vi "SetVoltage.vi"(3 "Voltage":dbl format="%.3f", 4 "error in":errorcluster, 5 "connection ID":refnum<k5>) -> (0 "False":bool, 1 "error out":errorcluster, 2 "connection ID out":refnum<k5>)   [LabVIEW 2013]
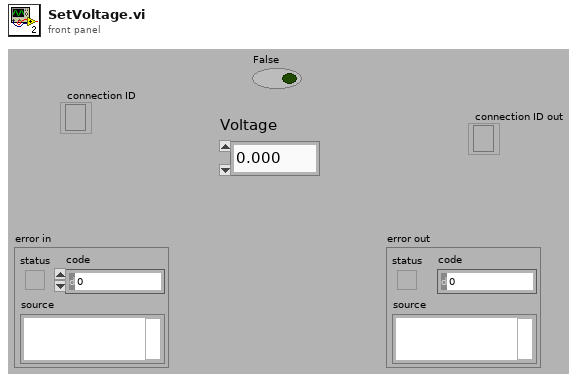
[diagram p1: front panel]
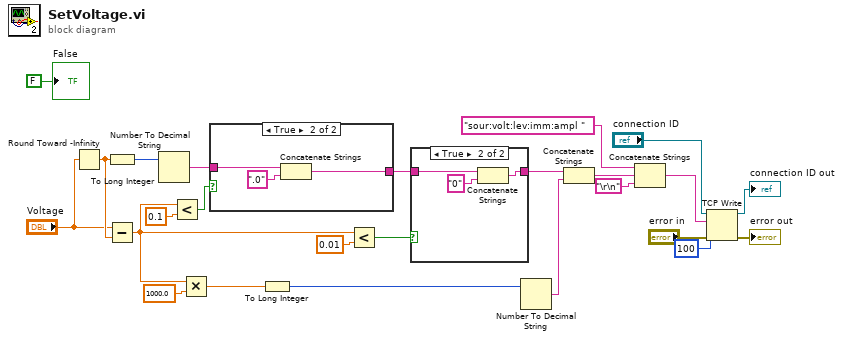
[diagram p0: block diagram]
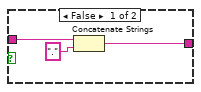
[diagram p3: hidden frame]
diagram:
  n1 = Round Toward -Infinity(1:"Voltage") -> (0:w17:dbl)
  n2 = To Long Integer(number=w17) -> (32bit integer=w15:i32)
  n3 = Subtract(x="Voltage", y=w17) -> (x-y=w10:dbl)
  n4 = Number To Decimal String(number=w15) -> (decimal integer string=w8:string)  [unwired: 1 out]
  n5 = Less?(x=w10, y=0.1) -> (x < y?=w9:bool)
  n6 = Multiply(x=w10, y=1000.0) -> (x*y=w18:dbl)
  n7 = case shown="True" w9 {
    tunnel: w8 -> [w27 w30]
    tunnel: [w26 w29] -> w6
    frame False {
      n8 = Concatenate Strings(w27, "." ("string")) -> (w26:string)
    }
    frame True {
      n9 = Concatenate Strings(w30, ".0" ("string")) -> (w29:string)
    }
  }
  n10 = To Long Integer(number=w18) -> (32bit integer=w16:i32)
  n11 = Less?(x=w10, y=0.01) -> (x < y?=w7:bool)
  n12 = case shown="True" w7 {
    tunnel: w6 -> [w32 w34]
    tunnel: [w32 w33] -> w5
    frame False {
    }
    frame True {
      n13 = Concatenate Strings(w34, "0" ("string")) -> (w33:string)
    }
  }
  n14 = Number To Decimal String(number=w16) -> (decimal integer string=w14:string)  [unwired: 1 out]
  n15 = Concatenate Strings(w5, w14) -> (w4:string)
  n16 = Concatenate Strings("sour:volt:lev:imm:ampl " ("data in"), w4, "\r\n") -> (w23:string)
  n17 = TCP Write(connection ID="connection ID", data in=w23, error in (no error)="error in", 9:100 ("timeout ms (25000)")) -> (connection ID out=→"connection ID out":refnum<k5>, error out=→"error out":errorcluster)  [unwired: 1 out]
  "False" <- FALSE
